vi "XY Graph Average Selected Plots Event.vi"(8 "Error In":errorcluster, 9 "Plots to ignore (none)":i32[](array[numeric]), 11 "XYGraph Ref":refnum<vi>) -> (0 "Error Out":errorcluster, 1 "Averaged Plot Names":string[](array[string]), 2 "Averaged Plot Indices":i32[](array[numeric]), 3 "Graph Label":string, 5 "Plot Name":string)   [LabVIEW 2021, in "XY Graph Add-Ons.lvlib"]
uses:
  XY Graph Add-Ons.lvlib
  f238f171-5771-4d28-99e7-c80d52bff377.vi
  XY Graph Add Single Plot with Name.vi
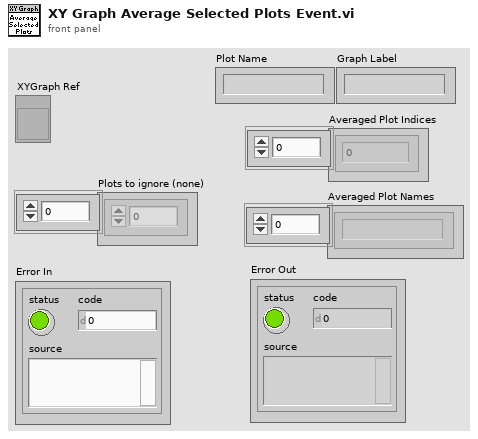
[diagram p1: front panel]
types:
  T1 = typedef "XY Graph Add-Ons.lvlib/XY Graph Refnum.ctl" = refnum<vi>
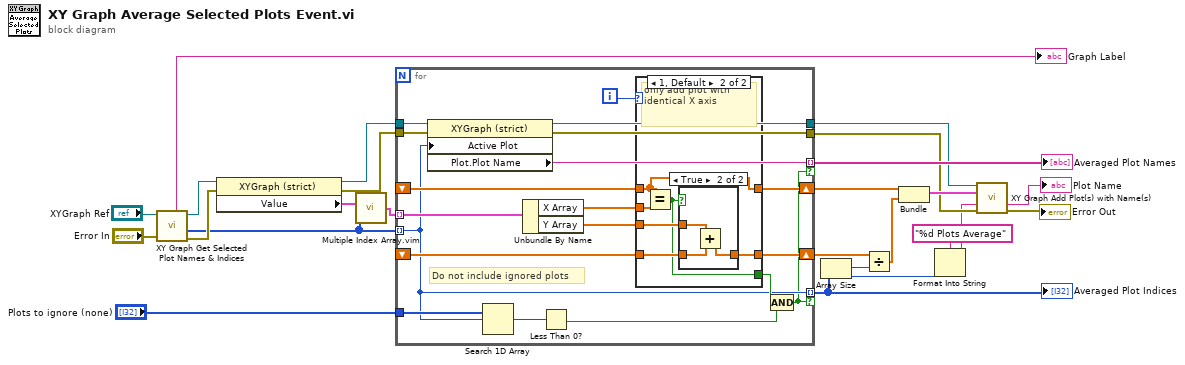
[diagram p0: block diagram]
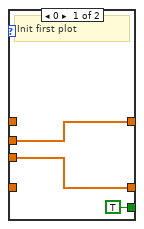
[diagram p2: hidden frame]
diagram:
  n1 = call "XY Graph Get Selected Plot Names & Indices.vi"("error in (no error)"="Error In", "XYGraph in"="XYGraph Ref") -> ("error out"=w21:errorcluster, "Selected Plots"=w3:i32[], "XYGraph out"=w22:T1, "Graph Name"=→"Graph Label":string)  [unwired: 5 in, 1 out]
  n2 = property class="XYGraph (strict)"(reference=w22, error in=w21) -> (reference out=w19:T1, error out=w15:errorcluster, "Value"=w2:cluster{"X Array":dbl[], "Y Array":dbl[]}[])
  n3 = call "Multiple Index Array.vim"("Index Array"=w3, "Array"=w2) -> ("Selected Element(s)"=w20:cluster{"X Array":dbl[], "Y Array":dbl[]}[])  [unwired: 4 in]
  n4 = for {
    tunnel: w20 -> [w43] mode=indexing
    shift-right: [w41] -> w14
    shift-left: _ -> [w38]
    shift-right: [w40] -> w16
    shift-left: _ -> [w37]
    tunnel: [w28] -> w17 mode=indexing if=w26
    tunnel: w19 -> [w36]
    tunnel: [w35] -> w18 mode=indexing if=w26
    tunnel: w15 -> [w33]
    tunnel: [w32] -> w10
    tunnel: [w31] -> w11
    tunnel: "Plots to ignore (none)" -> [w30]
    tunnel: w3 -> [w28] mode=indexing
    i -> [w29]
    # "Do not include ignored plots"
    n5 = property class="XYGraph (strict)"(reference=w36, error in=w33, "Active Plot"=w28) -> (reference out=w31:T1, error out=w32:errorcluster, "Plot.Plot Name"=w35:string)
    n6 = Search 1D Array(1D array=w30, element=w28) -> (index of element=w27:i32)  [unwired: 1 in]
    n7 = Unbundle By Name(w43) -> ("X Array"=w42:dbl[], "Y Array"=w39:dbl[])
    n8 = Less Than 0?(x=w27) -> (x < 0?=w25:bool)
    n9 = case shown="1, Default" w29 {
      tunnel: w42 -> [w46 w52]
      tunnel: [w46 w51] -> w41
      tunnel: [w45 w48] -> w40
      tunnel: w39 -> [w45 w50]
      tunnel: w38 -> [_ w51]
      tunnel: w37 -> [_ w49]
      tunnel: [TRUE w47] -> w34
      frame 0 {
        # "Init first plot"
      }
      frame 1, Default {
        # "only add plot with identical X axis"
        n10 = Equal?(x=w51, y=w52) -> (x = y?=w47:bool)
        n11 = case shown="True" w47 {
          tunnel: w50 -> [_ w56]
          tunnel: w49 -> [w53 w55]
          tunnel: [w53 w54] -> w48
          frame False {
          }
          frame True {
            n12 = Add(x=w56, y=w55) -> (x+y=w54:dbl[])
          }
        }
      }
    }
    n13 = Compound Arithmetic op=AND(w34, w25) -> (w26:bool)
  }
  "Averaged Plot Indices" <- w17
  "Averaged Plot Names" <- w18
  n14 = Array Size(array=w17) -> (size(s)=w9:i32)
  n15 = Divide(x=w16, y=w9) -> (x/y=w13:dbl[])
  n16 = Bundle("X Array"=w14, w13) -> (w12:cluster{"X Array":dbl[], dbl[]})  [unwired: 1 in]
  n17 = Format Into String(format string="%d Plots Average" ("initial string"), w9) -> (resulting string=w7:string)  [unwired: 2 in, 1 out]
  n18 = call-poly "XY Graph Add Plot(s) with Name(s).vi"("XYGraph Ref in"=w11, "Plot"=w12, "Plot Name (\"Plot\")"=w7, "error in (no error)"=w10) -> ("Plot Name"=→"Plot Name":string, "error out"=→"Error Out":errorcluster)  [unwired: 8 in, 2 out]
